vi "I2C Message Buffer - Enqueue.vi"(8 "error in (no error)":errorcluster, 11 "I2C Messages":string[][](array[string])) -> (0 "error out":errorcluster)   [LabVIEW 2025, in "I2C Bus Monitor.lvclass"]
uses:
  I2C Bus Monitor.lvclass
  Error Global.vi
  I2C Bus Monitor.lvclass/I2C Bus Monitor.ctl
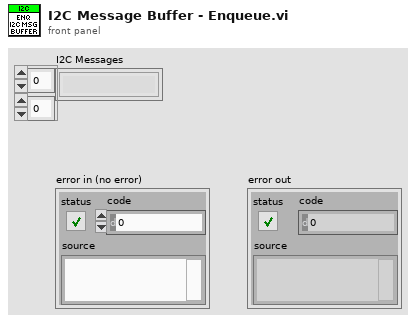
[diagram p1: front panel]
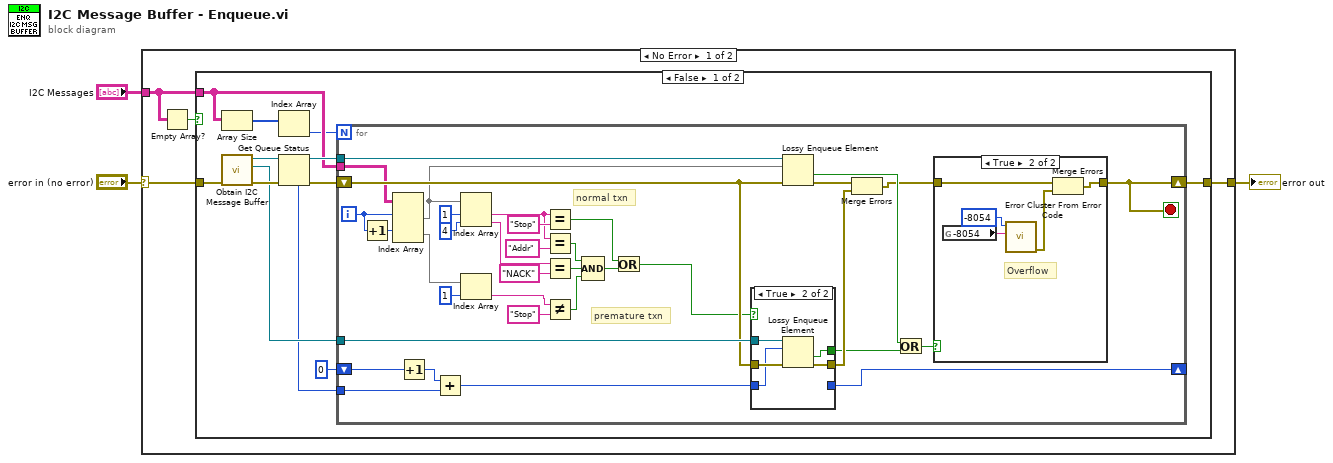
[diagram p0: block diagram]
diagram:
  n1 = case shown="No Error" "error in (no error)" {
    selector: "error in (no error)" -> [w6 w70]
    tunnel: [w7 w70] -> w3
    tunnel: "I2C Messages" -> [w4 _]
    frame No Error {
      n2 = Empty Array?(array=w4) -> (empty?=w5:bool)
      n3 = case shown="False" w5 {
        tunnel: [w19 w69] -> w7
        tunnel: w4 -> [w15 _]
        tunnel: w6 -> [w12 w69]
        frame False {
          n4 = Array Size(array=w15) -> (size(s)=w14:i32[])
          n5 = call "Obtain I2C Message Buffer.vi"("error in (no error)"=w12) -> ("error out"=w10:errorcluster, "Msgs per Txn Queue"=w9:refnum<queue>, "I2C Message Queue"=w11:refnum<queue>)  [unwired: 8 in]
          n6 = Index Array(array=w14) -> (element=w13:i32)  [unwired: 1 in]
          n7 = Get Queue Status(queue=w11, error in (no error)=w10) -> (queue out=w17:refnum<queue>, error out=w18:errorcluster, # elements in queue=w8:i32)  [unwired: 1 in, 5 out]
          n8 = for {
            N: w13 -> [_]
            tunnel: w17 -> [w54]
            tunnel: w15 -> [w35]
            shift-right: [w20] -> w19
            shift-left: w18 -> [w51]
            tunnel: w9 -> [w52]
            shift-right: [w47] -> _
            shift-left: 0 -> [w48]
            tunnel: w8 -> [w25]
            i -> [w33]
            stop <- w20 stop-if-true
            # "normal txn"
            # "premature txn"
            n9 = Increment(x=w33) -> (x+1=w32:i32)
            n10 = Index Array(array=w35, index (row) #1=w33, index (row) #2=w32) -> (element #1=w34:string[], element #2=w30:string[])  [unwired: 2 in]
            n11 = Increment(x=w48) -> (x+1=w46:i32)
            n12 = Add(x=w46, y=w25) -> (x+y=w26:i32)
            n13 = Index Array(array=w34, index #1=1 ("index"), index #2=4 ("index")) -> (element #1=w42:string, element #2=w37:string)
            n14 = Index Array(array=w30, index=1) -> (element=w28:string)
            n15 = Equal?(x=w42, y="Stop") -> (x = y?=w49:bool)
            n16 = Equal?(x=w42, y="Addr") -> (x = y?=w39:bool)
            n17 = Equal?(x=w37, y="NACK") -> (x = y?=w38:bool)
            n18 = Not Equal?(x=w28, y="Stop") -> (x != y?=w27:bool)
            n19 = Compound Arithmetic op=AND(w39, w38, w27) -> (w40:bool)
            n20 = Or(x=w49, y=w40) -> (x .or. y?=w43:bool)
            n21 = case shown="True" w43 {
              tunnel: w52 -> [_ w68]
              tunnel: w51 -> [w62 w67]
              tunnel: [w62 w66] -> w50
              tunnel: w26 -> [w63 w65]
              tunnel: [w63 _] -> w47
              tunnel: [_ w64] -> w22
              frame False {
              }
              frame True {
                n22 = Lossy Enqueue Element(queue=w68, element=w65, error in (no error)=w67) -> (overflow?=w64:bool, error out=w66:errorcluster)  [unwired: 2 out]
              }
            }
            n23 = Lossy Enqueue Element(queue=w54, element=w34, error in (no error)=w51) -> (overflow?=w23:bool, error out=w55:errorcluster)  [unwired: 2 out]
            n24 = Merge Errors(w55, w50) -> (w21:errorcluster)
            n25 = Or(x=w23, y=w22) -> (x .or. y?=w24:bool)
            n26 = case shown="True" w24 {
              tunnel: w21 -> [w56 w59]
              tunnel: [w56 w58] -> w20
              frame False {
              }
              frame True {
                # "Overflow"
                n27 = global read "Error Global.vi" "-8054"() -> (w61:string)
                n28 = call <vilib>:"Error Cluster From Error Code.vi"("error message (\"\")"=w61, "error code (0)"=-8054) -> ("error out"=w57:errorcluster)  [unwired: 7 in]
                n29 = Merge Errors(w59, w57) -> (w58:errorcluster)
              }
            }
          }
        }
        frame True {
        }
      }
    }
    frame Error {
    }
  }
  "error out" <- w3
